vi "sub_torad.vi"(11 "ヵ":dbl) -> (3 "rad":dbl)   [LabVIEW 2019]
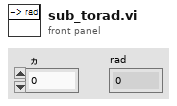
[diagram p1: front panel]
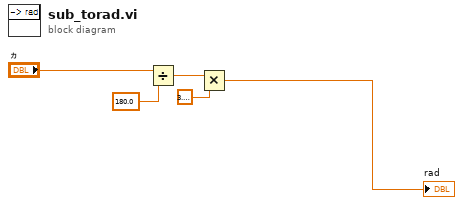
[diagram p0: block diagram]
diagram:
  n1 = Divide(x="ヵ", y=180.0) -> (x/y=w1:dbl)
  n2 = Multiply(x=w1, y=3.141592653589793) -> (x*y=→"rad":dbl)
